vi "Read AcknowledgeMsg.vi"(8 "error in (no error)":errorcluster, 11 "AsynchReturnMsg in":refnum<class "CS++AsynchReturnMsg.lvclass">) -> (0 "error out":errorcluster, 2 "AcknowledgeMsg":refnum<class "CS++AcknowledgeMsg.lvclass">, 3 "AsynchReturnMsg out":refnum<class "CS++AsynchReturnMsg.lvclass">)   [LabVIEW 2016, in "CS++AsynchReturnMsg.lvlib" / "CS++AsynchReturnMsg.lvclass"]
uses:
  CS++AsynchReturnMsg.lvclass
  CS++AcknowledgeMsg/CS++AcknowledgeMsg.lvclass
  CS++AsynchReturnMsg.lvclass/CS++AsynchReturnMsg.ctl
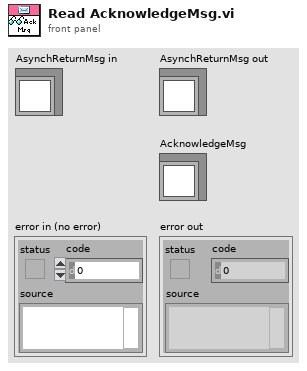
[diagram p1: front panel]
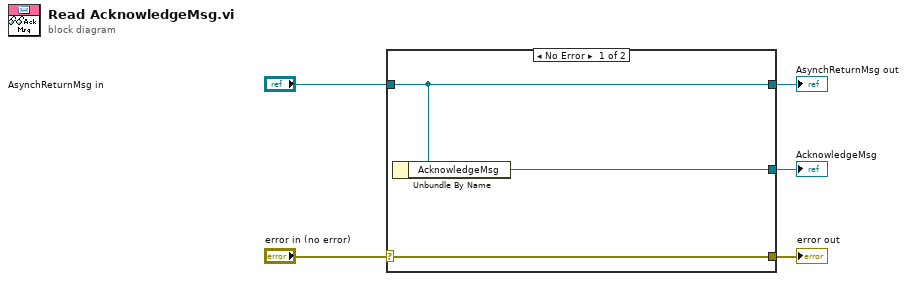
[diagram p0: block diagram]
diagram:
  n1 = case shown="No Error" "error in (no error)" {
    selector: "error in (no error)" -> [w8 w9]
    tunnel: [w8 w9] -> w4
    tunnel: [w7 w10] -> w2
    tunnel: "AsynchReturnMsg in" -> [w7 w10]
    tunnel: [w6 _] -> w1
    frame No Error {
      n2 = Unbundle By Name(w7) -> ("AcknowledgeMsg"=w6:refnum<class "CS++AcknowledgeMsg.lvclass">)
    }
    frame Error {
    }
  }
  "error out" <- w4
  "AsynchReturnMsg out" <- w2
  "AcknowledgeMsg" <- w1
